vi "Get VI Inputs and Outputs [String].vi"(8 "error in (no error)":errorcluster, 11 "VI Refnum":refnum<vi>) -> (0 "error out":errorcluster, 1 "VI Name":string, 2 "Outputs[]":cluster{"Name":string, "Value":string}[](array[cluster]), 3 "Inputs[]":cluster{"Name":string, "Value":string}[](array[cluster]))   [LabVIEW 2016, in "SLL Application.lvlib"]
doc: "Get the list of controls and indicators of a given VI reference, where values are converted to JSON string representation.\n\nIf the VI refnum input is not passed or invalid, it will automatically get the refnum of caller VI and use."
uses:
  SLL Application.lvlib
  <vilib>/addons/_JKI.lib/Serialization/JSON/JKI JSON Serialization.lvlib
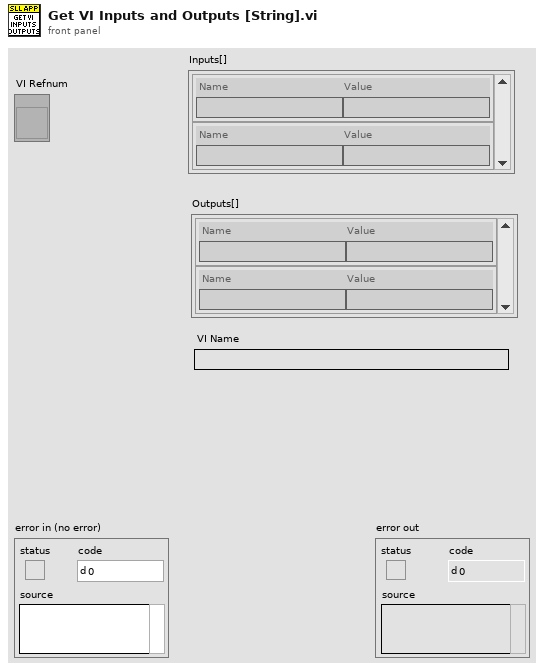
[diagram p1: front panel]
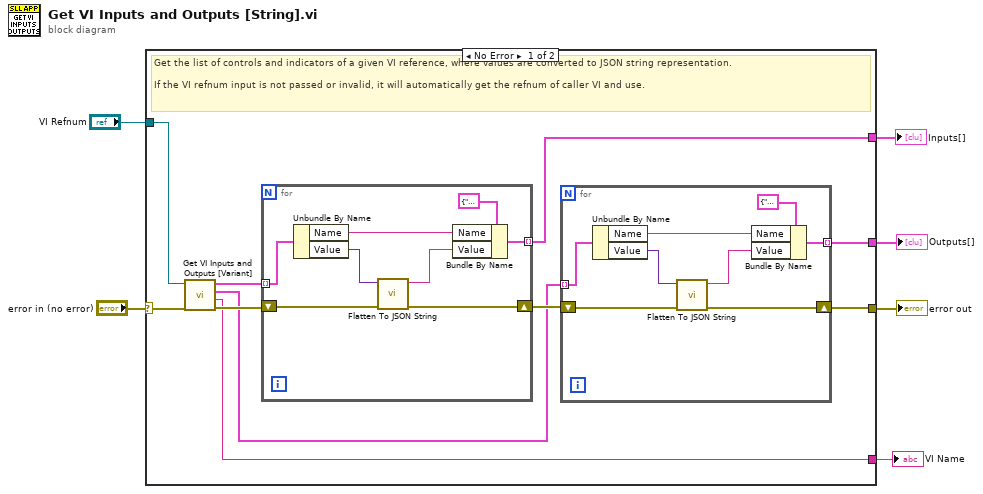
[diagram p0: block diagram]
diagram:
  n1 = case shown="No Error" "error in (no error)" {
    selector: "error in (no error)" -> [w16 w33]
    tunnel: [w8 w33] -> w5
    tunnel: "VI Refnum" -> [w15 _]
    tunnel: [w10 _] -> w3
    tunnel: [w9 _] -> w2
    tunnel: [w7 _] -> w1
    frame No Error {
      # "Get the list of controls and indicators of a given VI reference, where values are converted to JSON string representation.\n\nIf the VI refnum input is not passed or invalid, it will automatically get the refnum of caller VI and use."
      n2 = call "Get VI Inputs and Outputs [Variant].vi"("error in (no error)"=w16, "VI Refnum"=w15) -> ("error out"=w14:errorcluster, "VI Name"=w7:string, "Outputs[]"=w11:cluster{"Name":string, "Value":variant}[], "Inputs[]"=w13:cluster{"Name":string, "Value":variant}[])  [unwired: 6 in]
      n3 = for {
        tunnel: w13 -> [w32] mode=indexing
        tunnel: [w25] -> w10 mode=indexing
        shift-right: [w29] -> w12
        shift-left: w14 -> [w31]
        n4 = Unbundle By Name(w32) -> ("Name"=w27:string, "Value"=w30:variant)
        n5 = call <vilib>:"Flatten To JSON String.vi"("error in (no error)"=w31, "Variant"=w30) -> ("error out"=w29:errorcluster, "JSON String"=w26:string)  [unwired: 8 in]
        n6 = Bundle By Name(cluster=cluster{"Name":string, "Value":string} {"Name"="", "Value"=""} ("System Cluster"), "Name"=w27, "Value"=w26) -> (w25:cluster{"Name":string, "Value":string})
      }
      n7 = for {
        tunnel: w11 -> [w24] mode=indexing
        tunnel: [w17] -> w9 mode=indexing
        shift-right: [w21] -> w8
        shift-left: w12 -> [w23]
        n8 = Unbundle By Name(w24) -> ("Name"=w19:string, "Value"=w22:variant)
        n9 = call <vilib>:"Flatten To JSON String.vi"("error in (no error)"=w23, "Variant"=w22) -> ("error out"=w21:errorcluster, "JSON String"=w18:string)  [unwired: 8 in]
        n10 = Bundle By Name(cluster=cluster{"Name":string, "Value":string} {"Name"="", "Value"=""} ("System Cluster"), "Name"=w19, "Value"=w18) -> (w17:cluster{"Name":string, "Value":string})
      }
    }
    frame Error {
    }
  }
  "error out" <- w5
  "Inputs[]" <- w3
  "Outputs[]" <- w2
  "VI Name" <- w1
